vi "visionTarget.vi"(1 "Image":T1) -> (4 "Number of Particles (Particle Analysis 3)":i32, 6 "Distance to center of target":dbl, 8 "Image Out":T1(plugin-control), 10 "Distance across ground to wall":dbl, 15 "error out":errorcluster)   [LabVIEW 2012]
uses:
  <vilib>/vision/Image Controls.llb/IMAQ Image.ctl
  <vilib>/vision/NI_Vision_Development_Module.lvlib
panel:
  in  "Camera angle":dbl
  in  "Blue or Luma or Val or Inten Range":cluster{"Lower value":i32, "Upper value":i32}={"Lower value"=14, "Upper value"=255}
  in  "Green or Sat Range":cluster{"Lower value":i32, "Upper value":i32}={"Lower value"=148, "Upper value"=255}
  in  "Red or Hue Range":cluster{"Lower value":i32, "Upper value":i32}={"Lower value"=0, "Upper value"=255}
  in  "Left Motor":dbl
  in  "Right Motor":dbl
  out "Left Motor New":dbl
  out "Right Motor New":dbl
  in  "Degrees off center":dbl
  in  "height of camera off ground":dbl
  out "Particle Measurements (Pixels) (Particle Analysis 3)":dbl[][](array[numeric]) format="%.2f"
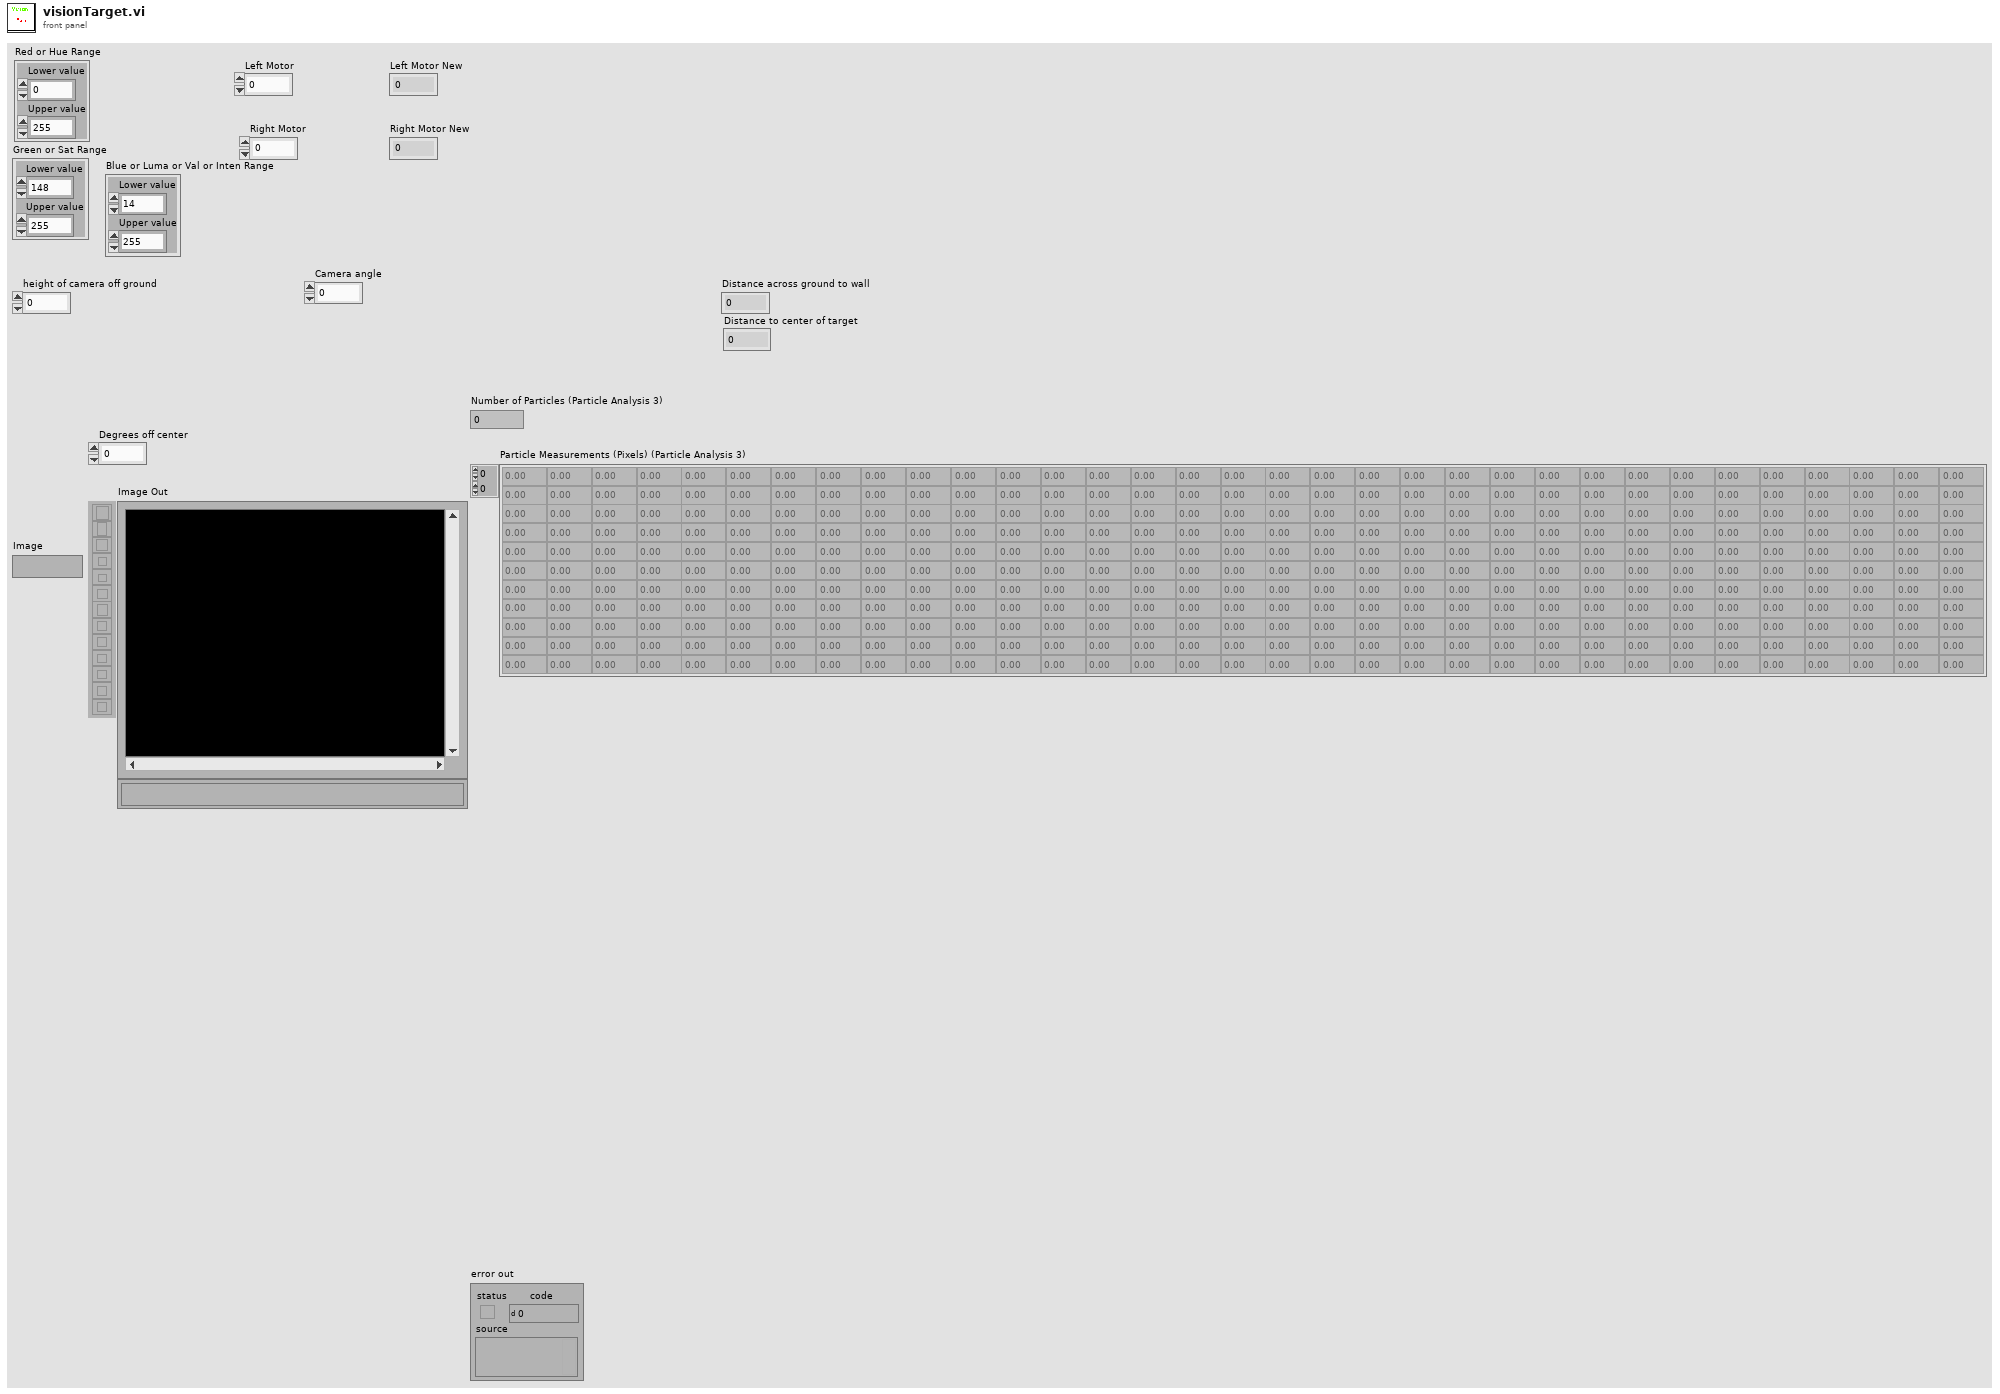
[diagram p1: front panel]
types:
  T1 = typedef "IMAQ Image.ctl" = refnum<image>
  T2 = typedef "Image Type" = u32
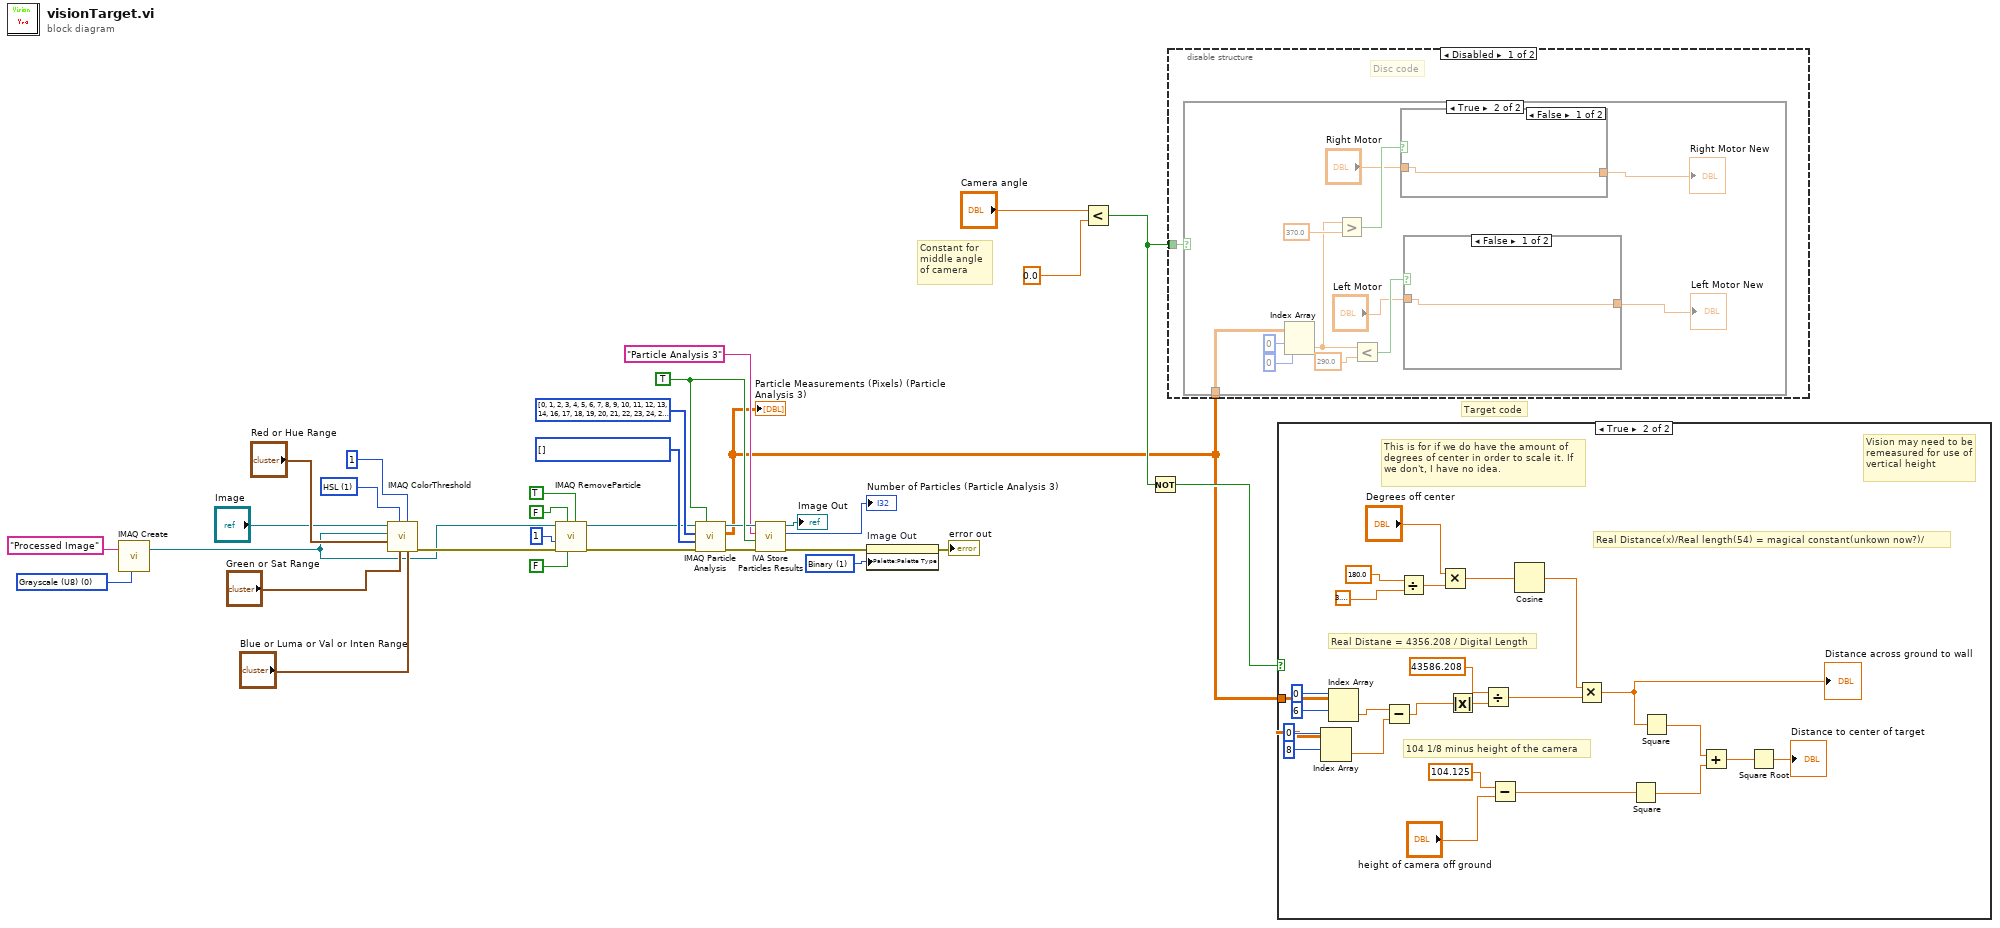
[diagram p0: block diagram]
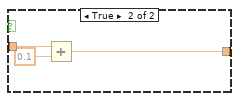
[diagram p3: hidden frame]
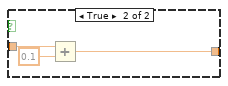
[diagram p4: hidden frame]
diagram:
  w3 = T2 0 items=["Grayscale (U8)", "Grayscale (I16)", "Grayscale (SGL)", "Complex (CSG)", "RGB (U32)", "HSL (U32)", "RGB (U64)"] ("Image Type")
  w13 = u32 1 items=["Grayscale", "Binary", "Gradient", "Rainbow", "Temperature", "User Defined"] ("Palette")
  w21 = i32[] [] items=["Center of Mass X", "Center of Mass Y", "First Pixel X", "First Pixel Y", "Bounding Rect Left", "Bounding Rect Top", "Bounding Rect Right", "Bounding Rect Bottom", "Max Feret Diameter Start X", "Max Feret Diameter Start Y", "Max Feret Diameter End X", "Max Feret Diameter End Y", "Max Horiz. Segment Length Left", "Max Horiz. Segment Length Right", "Max Horiz. Segment Length Row", "-", "Bounding Rect Width", "Bounding Rect Height", "Bounding Rect Diagonal", "Perimeter", "Convex Hull Perimeter", "Holes' Perimeter", "Max Feret Diameter", "Equivalent Ellipse Major Axis", "Equivalent Ellipse Minor Axis", "Equivalent Ellipse Minor Axis (Feret)", "Equivalent Rect Long Side", "Equivalent Rect Short Side", "Equivalent Rect Diagonal", "Equivalent Rect Short Side (Feret)", "Average Horiz. Segment Length", "Average Vert. Segment Length", "Hydraulic Radius", "Waddel Disk Diameter", "-", "Area", "Holes' Area", "Particle & Holes' Area", "Convex Hull Area", "Image Area", "-", "Number of Holes", "Number of Horiz. Segments", "Number of Vert. Segments", "-", "Orientation", "Max Feret Diameter Orientation", "-", "% Area/Image Area", "% Area/(Particle & Holes' Area)", "Ratio of Equivalent Ellipse Axes", "Ratio of Equivalent Rect Sides", "-", "Elongation Factor", "Compactness Factor", "Heywood Circularity Factor", "Type Factor", "-", "Sum X", "Sum Y", "Sum XX", "Sum XY", "Sum YY", "Sum XXX", "Sum XXY", "Sum XYY", "Sum YYY", "-", "Moment of Inertia XX", "Moment of Inertia XY", "Moment of Inertia YY", "Moment of Inertia XXX", "Moment of Inertia XXY", "Moment of Inertia XYY", "Moment of Inertia YYY", "Norm. Moment of Inertia XX", "Norm. Moment of Inertia XY", "Norm. Moment of Inertia YY", "Norm. Moment of Inertia XXX", "Norm. Moment of Inertia XXY", "Norm. Moment of Inertia XYY", "Norm. Moment of Inertia YYY", "Hu Moment 1", "Hu Moment 2", "Hu Moment 3", "Hu Moment 4", "Hu Moment 5", "Hu Moment 6", "Hu Moment 7"] ("Real-World Measurements")
  w22 = i32[] [0, 1, 2, 3, 4, 5, 6, 7, 8, 9, 10, 11, 12, 13, 14, 16, 17, 18, 19, 20, 21, 22, 23, 24, 25, 26, 27, 28, 29, 30, 31, 32, 33, 35, 36, 37, 38, 39, 41, 42, 43, 45, 46, 48, 49, 50, 51, 53, 54, 55, 56, 58, 59, 60, 61, 62, 63, 64, 65, 66, 68, 69, 70, 71, 72, 73, 74, 75, 76, 77, 78, 79, 80, 81, 82, 83, 84, 85, 86, 87, 88] items=["Center of Mass X", "Center of Mass Y", "First Pixel X", "First Pixel Y", "Bounding Rect Left", "Bounding Rect Top", "Bounding Rect Right", "Bounding Rect Bottom", "Max Feret Diameter Start X", "Max Feret Diameter Start Y", "Max Feret Diameter End X", "Max Feret Diameter End Y", "Max Horiz. Segment Length Left", "Max Horiz. Segment Length Right", "Max Horiz. Segment Length Row", "-", "Bounding Rect Width", "Bounding Rect Height", "Bounding Rect Diagonal", "Perimeter", "Convex Hull Perimeter", "Holes' Perimeter", "Max Feret Diameter", "Equivalent Ellipse Major Axis", "Equivalent Ellipse Minor Axis", "Equivalent Ellipse Minor Axis (Feret)", "Equivalent Rect Long Side", "Equivalent Rect Short Side", "Equivalent Rect Diagonal", "Equivalent Rect Short Side (Feret)", "Average Horiz. Segment Length", "Average Vert. Segment Length", "Hydraulic Radius", "Waddel Disk Diameter", "-", "Area", "Holes' Area", "Particle & Holes' Area", "Convex Hull Area", "Image Area", "-", "Number of Holes", "Number of Horiz. Segments", "Number of Vert. Segments", "-", "Orientation", "Max Feret Diameter Orientation", "-", "% Area/Image Area", "% Area/(Particle & Holes' Area)", "Ratio of Equivalent Ellipse Axes", "Ratio of Equivalent Rect Sides", "-", "Elongation Factor", "Compactness Factor", "Heywood Circularity Factor", "Type Factor", "-", "Sum X", "Sum Y", "Sum XX", "Sum XY", "Sum YY", "Sum XXX", "Sum XXY", "Sum XYY", "Sum YYY", "-", "Moment of Inertia XX", "Moment of Inertia XY", "Moment of Inertia YY", "Moment of Inertia XXX", "Moment of Inertia XXY", "Moment of Inertia XYY", "Moment of Inertia YYY", "Norm. Moment of Inertia XX", "Norm. Moment of Inertia XY", "Norm. Moment of Inertia YY", "Norm. Moment of Inertia XXX", "Norm. Moment of Inertia XXY", "Norm. Moment of Inertia XYY", "Norm. Moment of Inertia YYY", "Hu Moment 1", "Hu Moment 2", "Hu Moment 3", "Hu Moment 4", "Hu Moment 5", "Hu Moment 6", "Hu Moment 7"] ("Pixel Measurements")
  w18 = TRUE ("Connectivity 4/8 (8)")
  w31 = u16 1 items=["RGB", "HSL", "HSV", "HSI"] ("Color Mode")
  # "Constant for middle angle of camera"
  # "Target code"
  n1 = call "IMAQ Create"("Image Name"="Processed Image", "Image Type"=w3) -> ("New Image"=w1:T1)  [unwired: 2 in, 2 out]
  n2 = call "IMAQ ColorThreshold"("Blue or Luma or Val or Inten Range"="Blue or Luma or Val or Inten Range", "Replace Value"=1, "Green or Sat Range"="Green or Sat Range", "Color Mode"=w31, "Red or Hue Range"="Red or Hue Range", "Image Dst"=w1, "Image Src"="Image") -> ("error out"=w23:errorcluster)  [unwired: 1 in, 3 out]
  n3 = call "IMAQ RemoveParticle"("Connectivity 4/8 (8)"=TRUE, "Low Pass/High Pass (Low)"=FALSE, "Square/Hexa (Square)"=FALSE, "error in (no error)"=w23, "Number of Erosion"=1, "Image Src"=w1) -> ("error out"=w20:errorcluster, "Image Dst Out"=w19:T1)  [unwired: 1 in, 3 out]
  n4 = call "IMAQ Particle Analysis"("Connectivity 4/8 (8)"=w18, "error in (no error)"=w20, "Real-World Measurements"=w21, "Pixel Measurements"=w22, "Image"=w19) -> ("error out"=w15:errorcluster, "Particle Measurements (Pixels)"=w6:dbl[][], "Image Out (duplicate)"=w17:T1)  [unwired: 4 out]
  "Particle Measurements (Pixels) (Particle Analysis 3)" <- w6
  n5 = call <vilib>:"IVA Store Particles Results.vi"("error in (no error)"=w15, "Connectivity 4/8 (8)"=w18, "Step Name"="Particle Analysis 3", "Image in"=w17) -> ("error out"=w12:errorcluster, "Number of Particles"=→"Number of Particles (Particle Analysis 3)":i32, "Image dup"=→"Image Out":T1)  [unwired: 5 out]
  n6 = property on="Image Out" class="ImageControl"(error in=w12, "Palette:Palette Type"=w13) -> (error out=→"error out":errorcluster)  [unwired: 1 in, 1 out]
  n7 = Less?(x="Camera angle", y=0.0) -> (x < y?=w7:bool)
  n8 = Not(x=w7) -> (.not. x?=w8:bool)
  n9 = disable-structure shown="Disabled" {
    disable-tunnel: w7 -> [w34 _]
    disable-tunnel: w6 -> [w33 _]
    frame Disabled {
      # "Disc code"
      n10 = case shown="True" w34 {
        tunnel: w33 -> [_ w35]
        frame False {
        }
        frame True {
          n11 = Index Array(array=w35, index (row)=0, index (col)=0 ("disabled index (col)")) -> (element=w41:dbl)
          n12 = Greater?(x=w41, y=370.0) -> (0:w45:bool)
          n13 = Less?(x=w41, y=290.0) -> (x < y?=w46:bool)
          n14 = case shown="False" w45 {
            tunnel: "Right Motor" -> [w51 w54]
            tunnel: [w51 w53] -> w43
            frame False {
            }
            frame True {
              n15 = Add(x=w54, y=0.1) -> (x+y=w53:dbl)
            }
          }
          "Right Motor New" <- w43
          n16 = case shown="False" w46 {
            tunnel: "Left Motor" -> [w47 w50]
            tunnel: [w47 w49] -> w44
            frame False {
            }
            frame True {
              n17 = Add(x=w50, y=0.1) -> (x+y=w49:dbl)
            }
          }
          "Left Motor New" <- w44
        }
      }
    }
    frame Enabled {
    }
  }
  n18 = case shown="True" w8 {
    tunnel: w6 -> [_ w57]
    frame False {
    }
    frame True {
      # "Real Distance(x)/Real length(54) = magical constant(unkown now?)/"
      # "Vision may need to be remeasured for use of vertical height"
      # "This is for if we do have the amount of degrees of center in order to scale it. If we don't, I have no idea."
      # "104 1/8 minus height of the camera"
      # "Real Distane = 4356.208 / Digital Length"
      n19 = Index Array(array=w57, index (row)=8, index (col)=0 ("disabled index (col)")) -> (element=w76:dbl)
      n20 = Index Array(array=w57, index (row)=6, index (col)=0 ("disabled index (col)")) -> (element=w77:dbl)
      n21 = Subtract(x=w77, y=w76) -> (x-y=w75:dbl)
      n22 = Divide(x=180.0, y=3.141592653589793) -> (x/y=w61:dbl)
      n23 = Multiply(x="Degrees off center", y=w61) -> (x*y=w56:dbl)
      n24 = Absolute Value(x=w75) -> (abs(x)=w71:dbl)
      n25 = Divide(x=43586.208, y=w71) -> (x/y=w59:dbl)
      n26 = Subtract(x=104.125, y="height of camera off ground") -> (x-y=w64:dbl)
      n27 = Cosine(x=w56) -> (cos(x)=w55:dbl)
      n28 = Multiply(x=w55, y=w59) -> (x*y=w58:dbl)
      "Distance across ground to wall" <- w58
      n29 = Square(x=w64) -> (x^2=w69:dbl)
      n30 = Square(x=w58) -> (x^2=w70:dbl)
      n31 = Add(x=w70, y=w69) -> (x+y=w68:dbl)
      n32 = Square Root(x=w68) -> (sqrt(x)=→"Distance to center of target":dbl)
    }
  }
